vi "Configure Generator Dual Tone Signal.vi"(6 "Ratio (0.0)":dbl format="%^.3e", 7 "Frequency (0Hz)":dbl format="%#.9p", 8 "error in (no error)":errorcluster, 9 "Source (1)":i32=1 format="%.0g", 10 "Instance (1)":i32=1 format="%.0g", 11 "VISA resource name":refnum<visa-resource-name>) -> (0 "error out":errorcluster, 3 "VISA resource name out":refnum<visa-resource-name>)   [LabVIEW 2015, in "Rohde&Schwarz CMXP GPRF.lvlib"]
doc: "Defines dual tone modulation parameters\n\nAttributes:\nRSCMXPGPRF_ATTR_DUAL_TONE_FREQUENCY\nRSCMXPGPRF_ATTR_DUAL_TONE_RATIO\n\nRemote-control commands:\nSOURce:GPRF:GEN<i>:DTONe:OFRequency<source>\nSOURce:GPRF:GEN<i>:DTONe:RATio"
uses:
  <instrlib>/Rohde&Schwarz CMXP GPRF/Rohde&Schwarz CMXP GPRF.lvlib
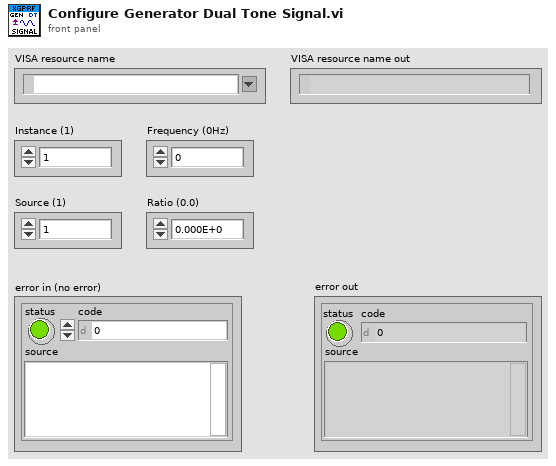
[diagram p1: front panel]
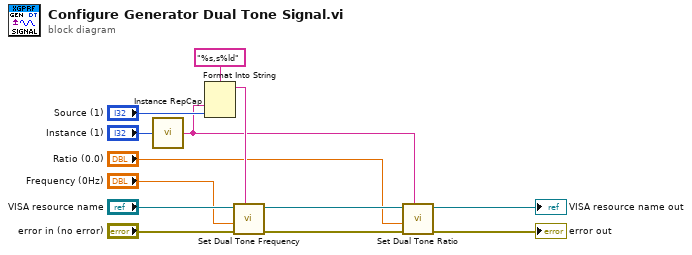
[diagram p0: block diagram]
diagram:
  n1 = call <instrlib>:"Instance RepCap.vi"("instance  in"="Instance (1)") -> ("instance out"=w3:string)
  n2 = Format Into String(format string="%s,s%ld", w3, "Source (1)") -> (resulting string=w5:string)  [unwired: 2 in, 1 out]
  n3 = call "Set Dual Tone Frequency"("Repeated Capabilities"=w5, "error in (no error)"="error in (no error)", "Dual Tone Frequency (0.0)"="Frequency (0Hz)", "instrument handle"="VISA resource name") -> ("error out"=w7:errorcluster, "instrument handle out"=w6:refnum<visa-resource-name>)  [unwired: 6 in]
  n4 = call "Set Dual Tone Ratio"("Repeated Capabilities"=w3, "error in (no error)"=w7, "Dual Tone Ratio (0.0)"="Ratio (0.0)", "instrument handle"=w6) -> ("error out"=→"error out":errorcluster, "instrument handle out"=→"VISA resource name out":refnum<visa-resource-name>)  [unwired: 6 in]
